vi "Write FIFO (Two Channels).vi"(0 "data in":u32[](array[numeric]), 1 "fifo 0":refnum<k21>, 2 "fifo 1":refnum<k21>, 5 "enable":bool[](array[boolean]), 9 "input valid":bool) -> (14 "ready for input":bool)   [LabVIEW 2016]
doc: "Writes data to two 32-bit FIFOs. This VI is a wrapper around the LabVIEW FPGA FIFO Write method. This VI exposes handshaking signals that inform the user when the FIFOs are ready to accept new data.\n\n<B>Input Parameters</B>\n\n<B>data in</B> is the data to be written to the FIFO.\n\n<B>enabled</B> specifies which streams are enabled.\n\n<B>input valid</B> specifies when 'data in' is valid.\n\n<B>reset</B> the LabVIEW FPGA FIFO.\n\n<B>fifo 0</B> is the reference to the FIFO to which data received on channel 0 will be written to.\n\n<B>fifo 1</B> is the reference to the FIFO to which data received on channel 1 will be written to.\n\n<B>Output Parameters</B>\n\n<B>ready for input</B> is a flow control signal that indicates whether the Write FIFO VI is ready to accept new data."
uses:
  <vilib>/rvi/DataTransferAndStorage/Container/XNode/niFpgaContainer.xnode
  <vilib>/rvi/FIFO/Fifo_Resource/niFpgaFifoEmulationRefIn.vi
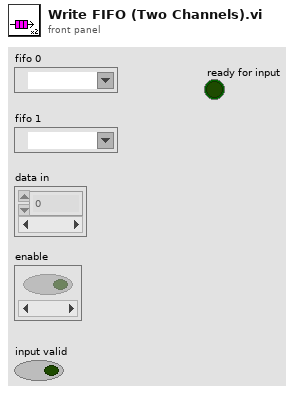
[diagram p1: front panel]
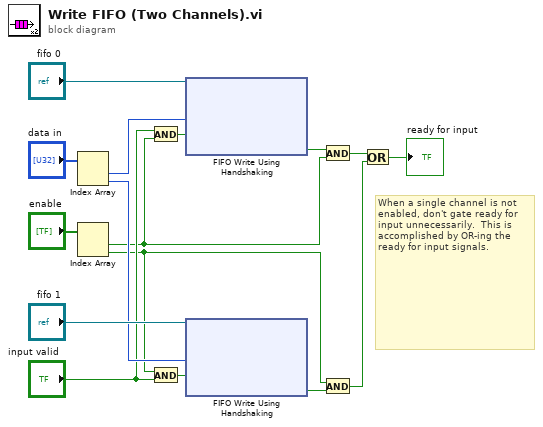
[diagram p0: block diagram]
diagram:
  # "When a single channel is not enabled, don't gate ready for input unnecessarily.  This is accomplished by OR-ing the ready for input signals."
  n1 = Index Array(array="data in") -> (element #1=w10:u32, element #2=w8:u32)  [unwired: 2 in]
  n2 = Index Array(array="enable") -> (element #1=w6:bool, element #2=w1:bool)  [unwired: 2 in]
  n3 = And(x="input valid", y=w6) -> (x .and. y?=w12:bool)
  n4 = And(x=w1, y="input valid") -> (x .and. y?=w9:bool)
  n5 = xnode "FIFO Write Using Handshaking"("Element"=w10, "Input Valid"=w12, "FIFO In"="fifo 0") -> ("Ready for Input"=w11:bool)  [unwired: 1 out]
  n6 = xnode "FIFO Write Using Handshaking"("FIFO In"="fifo 1", "Element"=w8, "Input Valid"=w9) -> ("Ready for Input"=w2:bool)  [unwired: 1 out]
  n7 = And(x=w11, y=w6) -> (x .and. y?=w5:bool)
  n8 = And(x=w1, y=w2) -> (x .and. y?=w4:bool)
  n9 = Or(x=w5, y=w4) -> (x .or. y?=→"ready for input":bool)
